vi "FTW-Test-Supervisor.vi"() -> (0 "Test Result":errorcluster)   [LabVIEW 2014]
uses:
  src/actor/supervisor/connector/FTW-Supervisor-Connector.lvclass
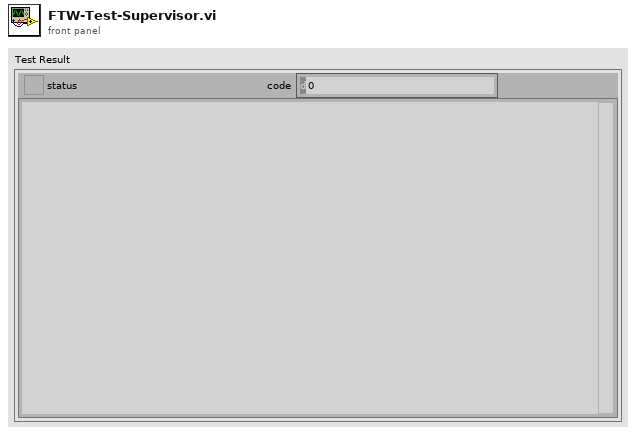
[diagram p1: front panel]
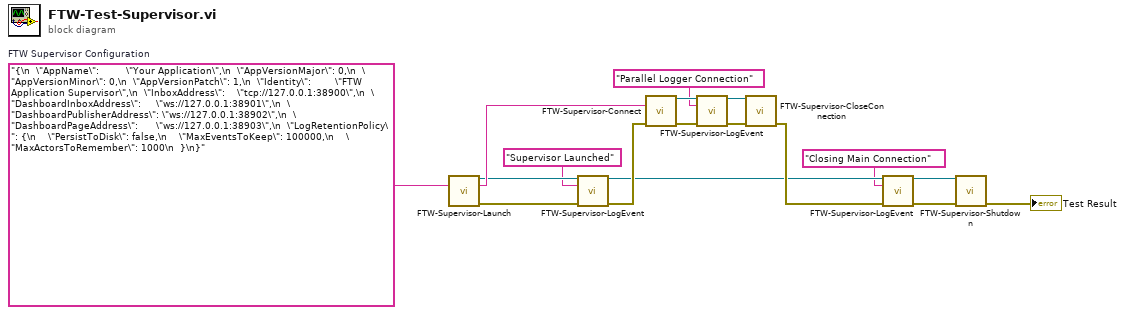
[diagram p0: block diagram]
diagram:
  w12 = "{\n  \"AppName\":         \"Your Application\",\n  \"AppVersionMajor\": 0,\n  \"AppVersionMinor\": 0,\n  \"AppVersionPatch\": 1,\n  \"Identity\":        \"FTW Application Supervisor\",\n  \"InboxAddress\":    \"tcp://127.0.0.1:38900\",\n  \"DashboardInboxAddress\":     \"ws://127.0.0.1:38901\",\n  \"DashboardPublisherAddress\": \"ws://127.0.0.1:38902\",\n  \"DashboardPageAddress\":      \"ws://127.0.0.1:38903\",\n  \"LogRetentionPolicy\": {\n    \"PersistToDisk\": false,\n    \"MaxEventsToKeep\": 100000,\n    \"MaxActorsToRemember\": 1000\n  }\n}"  # FTW Supervisor Configuration
  n1 = call "FTW-Supervisor-Launch.vi"("FTW Supervisor Configuration"=w12) -> ("FTW Supervisor Connection"=w11:refnum<class "FTW-Supervisor-Connector.lvclass">, "Supervisor Address"=w13:string, "error out"=w10:errorcluster)  [unwired: 12 in]
  n2 = call "FTW-Supervisor-LogEvent.vi"("FTW Supervisor Connection"=w11, "Event Type"="Supervisor Launched", "error in"=w10) -> ("FTW Supervisor Connection out"=w5:refnum<class "FTW-Supervisor-Connector.lvclass">, "error out"=w9:errorcluster)  [unwired: 11 in]
  n3 = call "FTW-Supervisor-Connect.vi"("Supervisor Address"=w13, "error in"=w9) -> ("FTW Supervisor Connection"=w16:refnum<class "FTW-Supervisor-Connector.lvclass">, "error out"=w14:errorcluster)  [unwired: 12 in]
  n4 = call "FTW-Supervisor-LogEvent.vi"("FTW Supervisor Connection"=w16, "Event Type"="Parallel Logger Connection", "error in"=w14) -> ("FTW Supervisor Connection out"=w7:refnum<class "FTW-Supervisor-Connector.lvclass">, "error out"=w6:errorcluster)  [unwired: 11 in]
  n5 = call "FTW-Supervisor-CloseConnection.vi"("FTW Supervisor Connection"=w7, "error in"=w6) -> ("error out"=w17:errorcluster)  [unwired: 13 in]
  n6 = call "FTW-Supervisor-LogEvent.vi"("FTW Supervisor Connection"=w5, "Event Type"="Closing Main Connection", "error in"=w17) -> ("FTW Supervisor Connection out"=w3:refnum<class "FTW-Supervisor-Connector.lvclass">, "error out"=w2:errorcluster)  [unwired: 11 in]
  n7 = call "FTW-Supervisor-Shutdown.vi"("FTW Supervisor Connection"=w3, "error in"=w2) -> ("error out"=→"Test Result":errorcluster)  [unwired: 13 in]
